vi "Initialize.vi"(8 "error in":errorcluster, 10 "Device":string) -> (0 "error out":errorcluster, 3 "Oven out":refnum<class "Oven.lvclass">)   [LabVIEW 2018, in "Oven.lvlib" / "Oven.lvclass"]
uses:
  Oven.lvclass
  Oven.lvclass/Oven.ctl
  PPLs/Configuration/Configuration.lvlibp/Configuration.lvclass
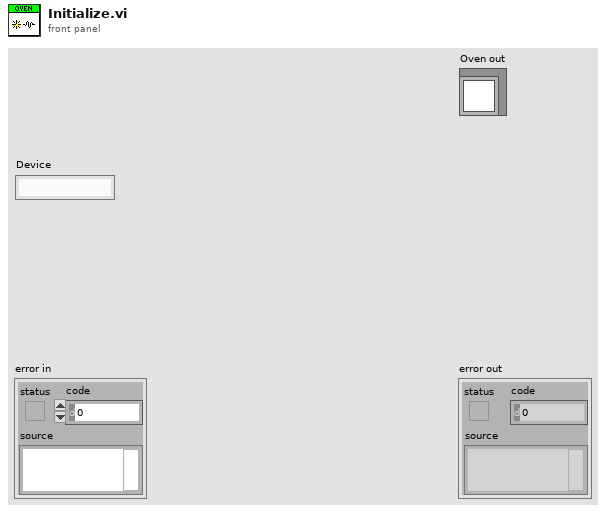
[diagram p1: front panel]
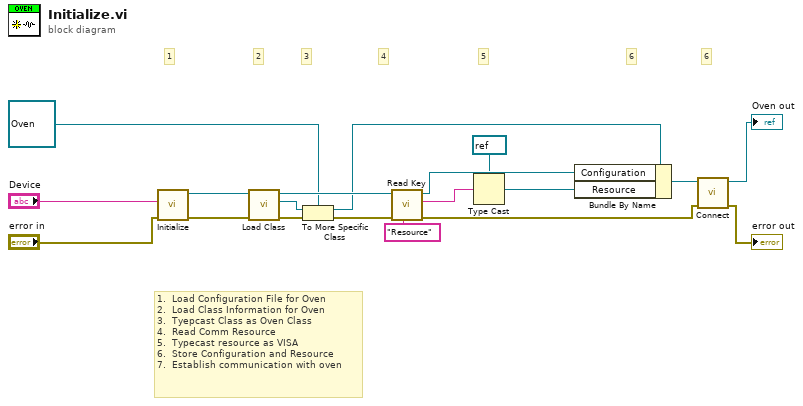
[diagram p0: block diagram]
diagram:
  # "1.  Load Configuration File for Oven\n2.  Load Class Information for Oven\n3.  Tyepcast Class as Oven Class\n4.  Read Comm Resource\n5.  Typecast resource as VISA\n6.  Store Configuration and Resource\n7.  Establish communication with oven"
  # "6"
  # "6"
  # "5"
  # "4"
  # "3"
  # "2"
  # "1"
  n1 = call "Initialize.vi"("error in"="error in", "Device"="Device") -> ("error out"=w17:errorcluster, "Configuration out"=w19:refnum<class "Configuration.lvclass">)  [unwired: 8 in]
  n2 = call "Load Class.vi"("error in"=w17, "Configuration in"=w19) -> ("error out"=w15:errorcluster, "Class out"=w14:refnum<class>, "Configuration out"=w18:refnum<class "Configuration.lvclass">)  [unwired: 7 in]
  n3 = To More Specific Class(target class=refnum<class "Oven.lvclass"> refnum ("Oven in"), reference=w14, error in=w15) -> (specific class reference=w12:refnum<class "Oven.lvclass">, error out=w7:errorcluster)
  n4 = call "Read Key.vi"("Key:"="Resource", "error in"=w7, "Configuration in"=w18) -> ("error out"=w4:errorcluster, "Value"=w10:string, "Configuration out"=w11:refnum<class "Configuration.lvclass">)  [unwired: 6 in]
  n5 = Type Cast(type=refnum<visa-resource-name> refnum ("Resource"), x=w10) -> (*(type *) &x=w8:refnum<visa-resource-name>)
  n6 = Bundle By Name(cluster=w12, "Configuration"=w11, "Resource"=w8) -> (w5:refnum<class "Oven.lvclass">)
  n7 = call-dynamic "Connect.vi"("error in (no error)"=w4, "Oven in"=w5) -> ("error out"=→"error out":errorcluster, "Oven out"=→"Oven out":refnum<class "Oven.lvclass">)  [unwired: 8 in]
